vi "REPORT - Autofrettage.vi"(8 "error in (no error)":errorcluster, 10 "Report Save Path":path, 11 "TDMS file path":path) -> ()   [LabVIEW 2025]
uses:
  <vilib>/printing/EasyPrintingControls.llb/contents.ctl
  <vilib>/Utility/NIReport.llb/Report Type (with Quick Print).ctl
  <vilib>/Utility/error.llb/Trim Whitespace One-Sided.vi
  <vilib>/printing/EasyPrinting.llb/Print VI Panel or Documentation (path).vi
  <vilib>/Utility/NIReport.llb/NI_report.lvclass
  <vilib>/Utility/NIReport.llb/NI_ReportGenerationCore.lvlib
panel:
  in  "Close":bool
  in  "PRINT REPORT":bool
  out "graph":cluster{"X":dbl[], "Y":dbl[]}[](graph)
  out "Operator:":string
  out "String":string
  in  "Comments:":string
  out "Test Date:":dbl format="%<%x>T"
  out "Test ID:":string
  out "Part Number:":string
  out "Job Number:":string
  # "Autofrettage Run Report"
  # "Unit Under Test"
  # "Pressure v. Time"
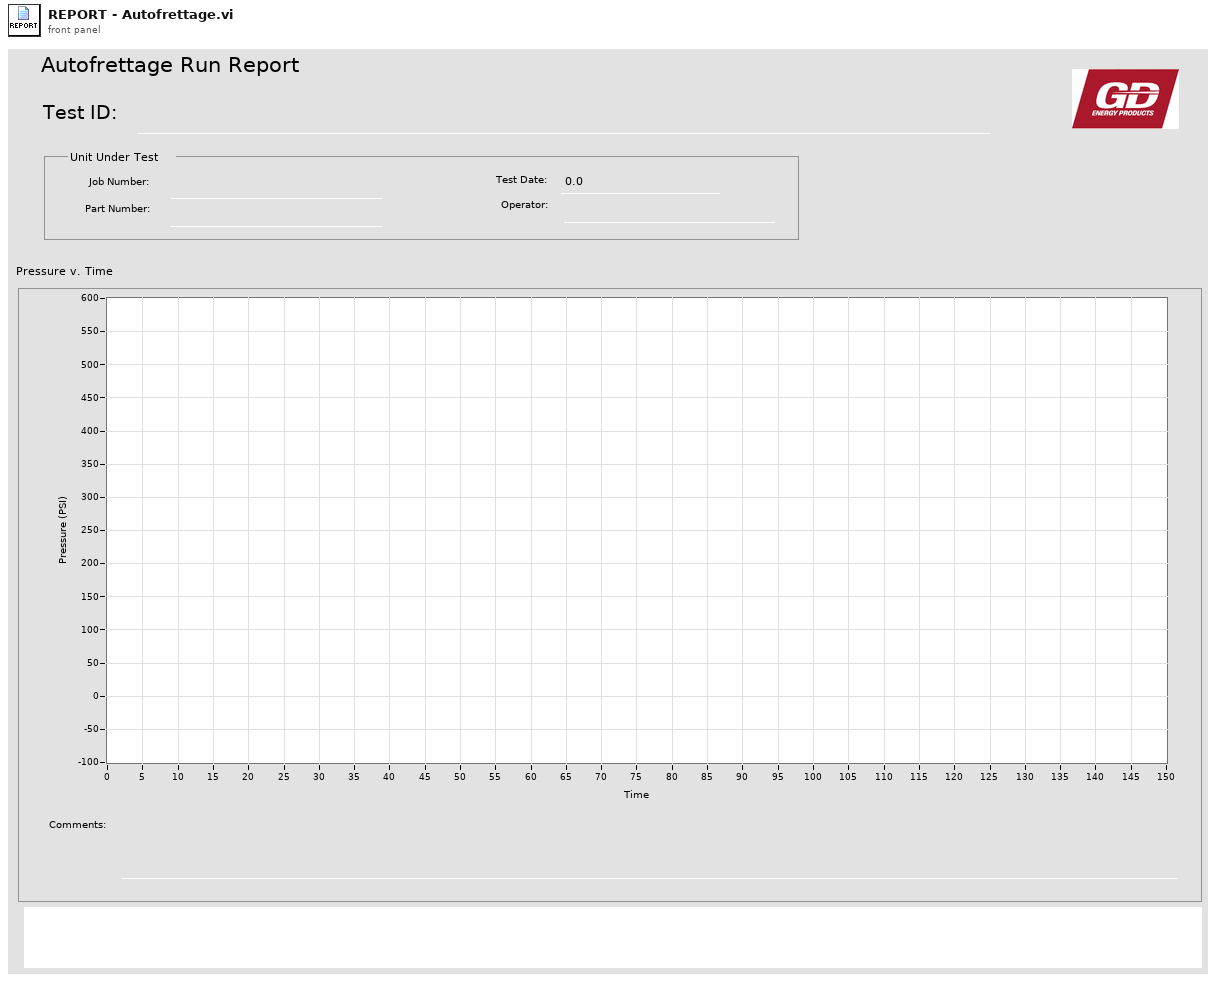
[diagram p1: front panel]
types:
  T1 = typedef "NI_ReportGenerationCore.lvlib/Report Type (with Quick Print).ctl" = enum16{"Quick Print", "HTML", "Word", "Excel"}
  T2 = typedef "NI_ReportGenerationCore.lvlib/contents.ctl" = u16
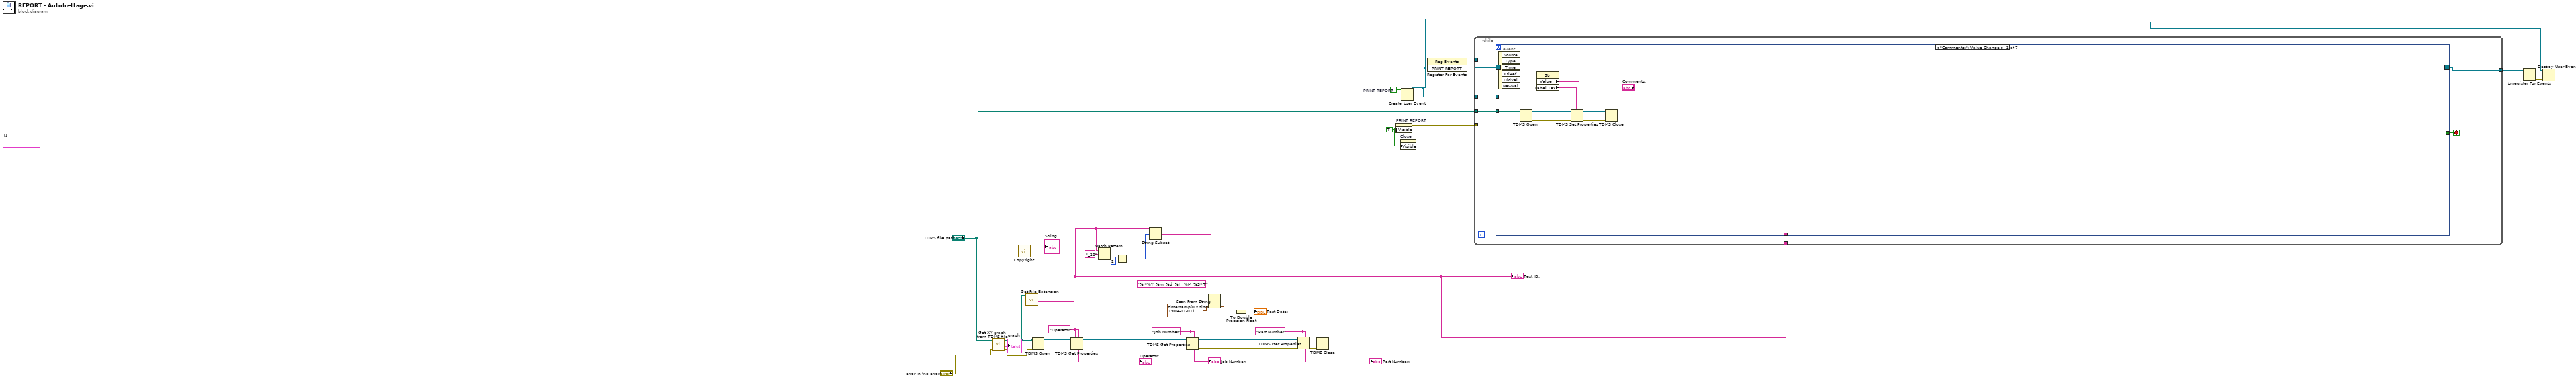
[diagram p0: block diagram]
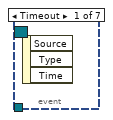
[diagram p2: hidden frame]
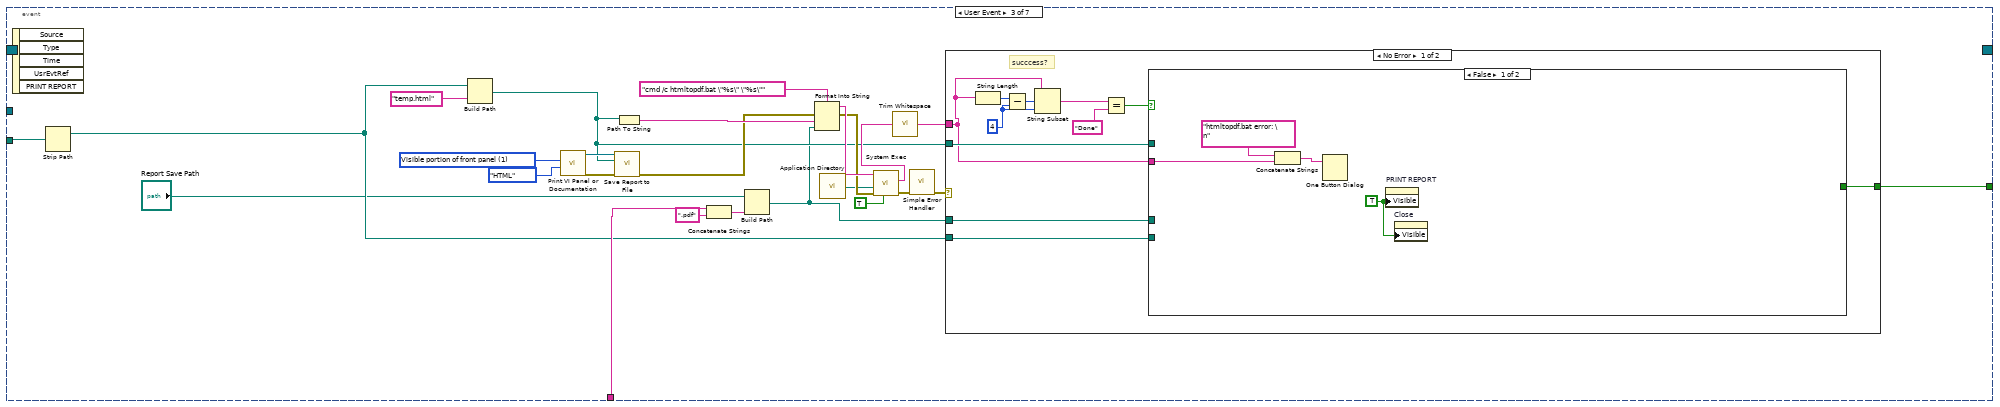
[diagram p3: hidden frame]
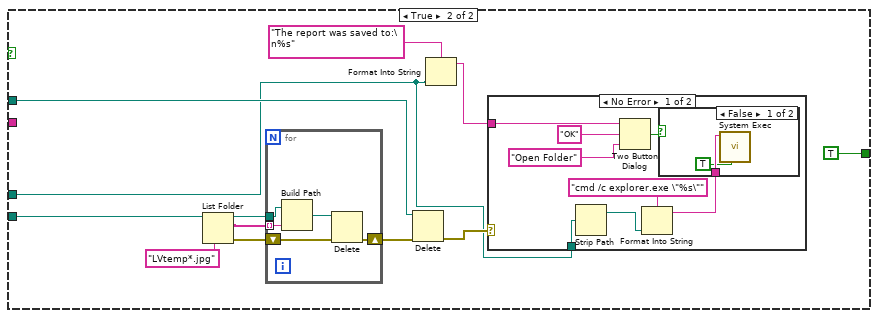
[diagram p4: hidden frame]
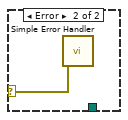
[diagram p6: hidden frame]
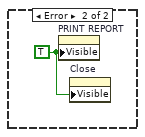
[diagram p7: hidden frame]
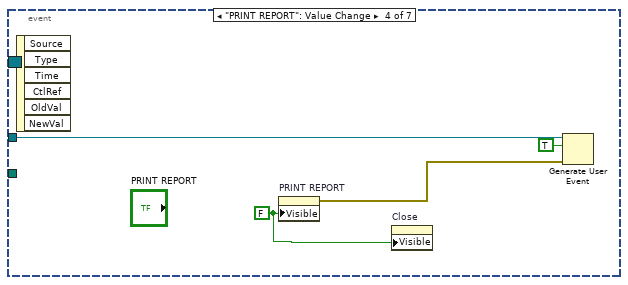
[diagram p8: hidden frame]
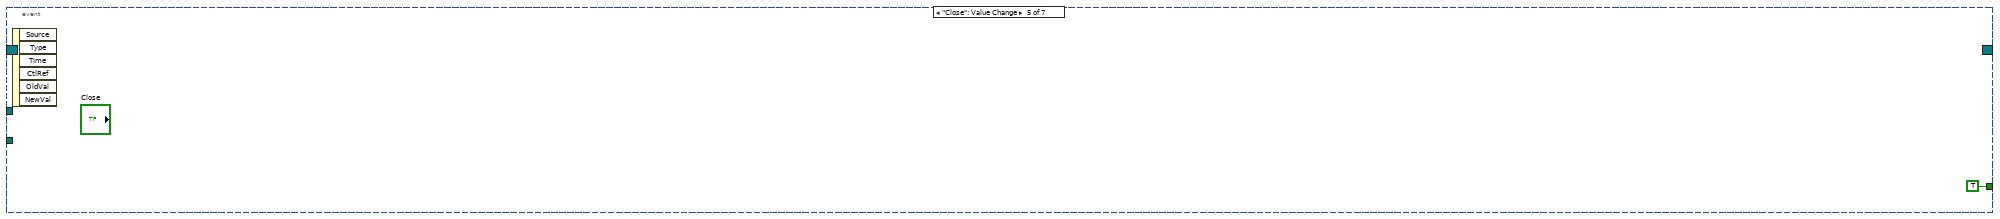
[diagram p9: hidden frame]
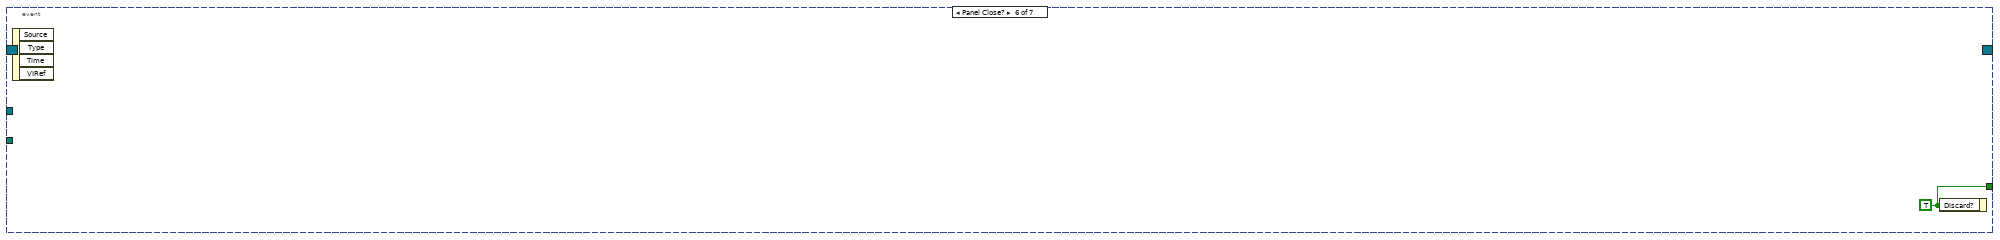
[diagram p10: hidden frame]
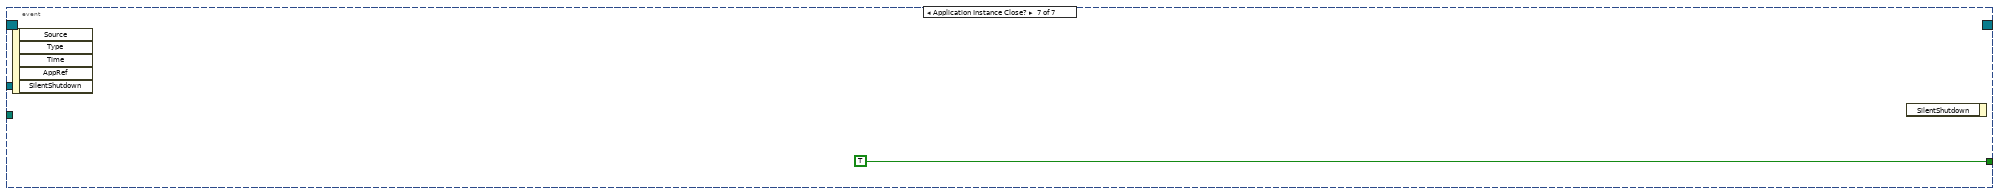
[diagram p11: hidden frame]
diagram:
  w10 = TRUE ("Visible")
  w16 = TRUE  # PRINT REPORT
  w23 = "Part Number" ("channel name")
  w25 = "Job Number" ("channel name")
  w21 = "Operator" ("channel name")
  (unwired) cluster{"X":dbl[], "Y":dbl[]}[] [] ("Restoring Force")
  n1 = call "Get XY graph from TDMS file.vi"("error in"="error in (no error)", "TDMS file path"="TDMS file path") -> ("error out"=w8:errorcluster, "graph"=→"graph":cluster{"X":dbl[], "Y":dbl[]}[], "TDMS file path out"=w7:path)  [unwired: 7 in]
  n2 = call "Copyright.vi"() -> ("String"=→"String":string)  [unwired: 11 in]
  n3 = call <vilib>:"Get File Extension.vi"("file"=w7) -> ("filename without extension"=w2:string)  [unwired: 6 in, 4 out]
  "Test ID:" <- w2
  n4 = TDMS Open(8:w8, 11:w7) -> (0:w30:errorcluster, 3:w35:refnum<k34>)  [unwired: 5 in]
  n5 = TDMS Get Properties(5:w21, 7:w21, 8:w30, 11:w35) -> (0:w31:errorcluster, 3:w34:refnum<k34>, 4:→"Operator:":string)  [unwired: 2 in, 3 out]
  n6 = Match Pattern(string=w2, regular expression="_20") -> (offset past match=w5:i32)  [unwired: 1 in, 3 out]
  n7 = Subtract(x=w5, y=2) -> (x-y=w3:i32)
  n8 = String Subset(string=w2, offset (0)=w3) -> (substring=w1:string)  [unwired: 1 in]
  n9 = TDMS Get Properties(5:w25, 7:w25, 8:w31, 11:w34) -> (0:w32:errorcluster, 3:w33:refnum<k34>, 4:→"Job Number:":string)  [unwired: 2 in, 3 out]
  n10 = Scan From String(format string="%<%Y_%m_%d_%H_%M_%S>T", input string=w1, default 1=timestamp(0 s since 1904-01-01)) -> (output 1=w27:timestamp)  [unwired: 2 in, 3 out]
  n11 = To Double Precision Float(number=w27) -> (double precision float=→"Test Date:":dbl)
  n12 = TDMS Get Properties(5:w23, 7:w23, 8:w32, 11:w33) -> (0:w18:errorcluster, 3:w17:refnum<k34>, 4:→"Part Number:":string)  [unwired: 2 in, 3 out]
  n13 = TDMS Close(8:w18, 11:w17) -> ()  [unwired: 2 out]
  n14 = property on="PRINT REPORT" class="Bool"("Visible"=w10) -> (error out=w11:errorcluster)  [unwired: 2 in, 1 out]
  n15 = property on="Close" class="Bool"("Visible"=w10) -> ()  [unwired: 2 in, 2 out]
  n16 = Create User Event(user event datatype=w16) -> (user event=w12:refnum<user-event>)  [unwired: 1 in, 1 out]
  n17 = register-events(w12) -> (reference out=w15:refnum<event-registration>)  [unwired: 2 in, 1 out]
  n18 = while {
    tunnel: "TDMS file path" -> [w42]
    tunnel: w2 -> [w41]
    tunnel: w15 -> [w40]
    tunnel: w12 -> [w39]
    tunnel: [w38] -> w14
    tunnel: w11 -> [_]
    stop <- w43 stop-if-true
    n19 = event shown="[1] \"Comments:\": Value Change" {
      selector: w40 -> [_ _ _ _ _ _ _]
      dyn-events: [_ _ _ _ _ _ _] -> w38
      timeout: _ -> [_ _ _ _ _ _ _]
      tunnel: [_ _ w73 _ TRUE ("Discard?") w126 TRUE] -> w43
      tunnel: w42 -> [_ w51 w75 _ _ _ _]
      tunnel: w41 -> [_ _ w76 _ _ _ _]
      tunnel: w39 -> [_ _ _ w124 _ _ _]
      event Timeout {
        n20 = event-data() -> ()  [unwired: 1 in, 3 out]
      }
      event "Comments:": Value Change {
        n21 = event-data() -> ("CtlRef"=w49:refnum<vi>)  [unwired: 1 in, 5 out]
        n22 = TDMS Open(11:w51) -> (0:w44:errorcluster, 3:w50:refnum<k34>)  [unwired: 6 in]
        n23 = property class="Str"(reference=w49) -> ("Value"=w46:string, "Label.Text"=w47:string)  [unwired: 1 in, 2 out]
        n24 = TDMS Set Properties(5:w46, 7:w47, 8:w44, 11:w50) -> (0:w45:errorcluster, 3:w48:refnum<k34>)  [unwired: 2 in, 2 out]
        n25 = TDMS Close(8:w45, 11:w48) -> ()  [unwired: 2 out]
      }
      event User Event {
        w67 = T2 1 items=["Complete front panel", "Visible portion of front panel", "Icon, description, panel and diagram", "Documentation: Using the panel", "Documentation: Using as a subVI", "Documentation: Complete", "Documentation: Custom"] ("contents (complete front panel)")
        n26 = event-data() -> ()  [unwired: 1 in, 5 out]
        n27 = Strip Path(path=w75) -> (stripped path=w74:path)  [unwired: 1 out]
        n28 = Build Path(base path=w74, name or relative path="temp.html" ("string")) -> (appended path=w56:path)
        n29 = call-poly <vilib>:"Print VI Panel or Documentation.vi"("report type (Quick Print)"=Report_Type_(with_Quick_Print)."HTML", "contents (complete front panel)"=w67) -> ("error out"=w64:errorcluster, "report out"=w70:refnum<class "NI_report.lvclass">)  [unwired: 8 in]
        n30 = call-dynamic "Save Report to File.vi"("report in"=w70, "report file path"=w56, "error in (no error)"=w64) -> ("error out"=w60:errorcluster)  [unwired: 11 in, 1 out]
        n31 = Path To String(path=w56) -> (string=w71:string)
        n32 = Concatenate Strings(w76, ".pdf" ("string")) -> (w62:string)
        n33 = Build Path(base path="Report Save Path", name or relative path=w62) -> (appended path=w54:path)
        n34 = Format Into String(format string="cmd /c htmltopdf.bat \"%s\" \"%s\"" ("command line"), error in=w60, w71, w54) -> (resulting string=w72:string, error out=w65:errorcluster)  [unwired: 1 in]
        n35 = call <vilib>:"Application Directory.vi"() -> ("Application Directory"=w55:path)
        n36 = call <vilib>:"System Exec.vi"("run minimized? (F)"=TRUE, "error in (no error)"=w65, "working directory"=w55, "command line"=w72) -> ("error out"=w66:errorcluster, "standard error"=w58:string)  [unwired: 4 in, 2 out]
        n37 = call <vilib>:"Trim Whitespace.vi"("string"=w58) -> ("trimmed string"=w52:string)  [unwired: 1 in]
        n38 = call <vilib>:"Simple Error Handler.vi"("error in (no error)"=w66) -> ("error out"=w59:errorcluster)  [unwired: 4 in, 4 out]
        n39 = case shown="No Error" w59 {
          tunnel: w74 -> [w87 _]
          tunnel: w56 -> [w86 _]
          tunnel: w52 -> [w77 _]
          tunnel: [w85 _] -> w73
          tunnel: w54 -> [w84 _]
          frame No Error {
            w81 = 4 ("y")
            # "succcess?"
            n40 = String Length(string=w77) -> (length=w83:i32)
            n41 = Subtract(x=w83, y=w81) -> (x-y=w82:i32)
            n42 = String Subset(string=w77, offset (0)=w82, length (rest)=w81) -> (substring=w80:string)
            n43 = Equal?(x=w80, y="Done") -> (x = y?=w78:bool)
            n44 = case shown="False" w78 {
              tunnel: w87 -> [_ w103]
              tunnel: w86 -> [_ w102]
              tunnel: w77 -> [w90 _]
              tunnel: [_ TRUE] -> w85
              tunnel: w84 -> [_ w97]
              frame False {
                w91 = TRUE ("Visible")
                n45 = Concatenate Strings("htmltopdf.bat error: \n" ("string"), w90) -> (w89:string)
                n46 = One Button Dialog(message=w89) -> ()  [unwired: 1 in, 1 out]
                n47 = property on="PRINT REPORT" class="Bool"("Visible"=w91) -> ()  [unwired: 2 in, 2 out]
                n48 = property on="Close" class="Bool"("Visible"=w91) -> ()  [unwired: 2 in, 2 out]
              }
              frame True {
                n49 = List Folder(path=w103, pattern="LVtemp*.jpg") -> (path out=w94:path, filenames=w95:string[], error out=w92:errorcluster)  [unwired: 2 in, 1 out]
                n50 = for {
                  tunnel: w95 -> [w108] mode=indexing
                  tunnel: w94 -> [w107]
                  shift-right: [w105] -> w93
                  shift-left: w92 -> [w104]
                  n51 = Build Path(base path=w107, name or relative path=w108) -> (appended path=w106:path)
                  n52 = Delete(path (use dialog)=w106, error in=w104) -> (error out=w105:errorcluster)  [unwired: 3 in, 2 out]
                }
                n53 = Delete(path (use dialog)=w102, error in=w93) -> (error out=w98:errorcluster)  [unwired: 3 in, 2 out]
                n54 = Format Into String(format string="The report was saved to:\n%s", w97) -> (resulting string=w99:string)  [unwired: 2 in, 1 out]
                n55 = case shown="No Error" w98 {
                  selector: w98 -> [_ w119]
                  tunnel: w99 -> [w116 _]
                  tunnel: w97 -> [w110 _]
                  frame No Error {
                    n56 = Strip Path(path=w110) -> (stripped path=w109:path)  [unwired: 1 out]
                    n57 = Two Button Dialog(message=w116, 1:"Open Folder" ("F button name (\"Cancel\")"), 2:"OK" ("T button name (\"OK\")")) -> (T button?=w114:bool)
                    n58 = Format Into String(format string="cmd /c explorer.exe \"%s\"", w109) -> (resulting string=w112:string)  [unwired: 2 in, 1 out]
                    n59 = case shown="False" w114 {
                      tunnel: w112 -> [w118 _]
                      frame False {
                        n60 = call <vilib>:"System Exec.vi"("run minimized? (F)"=TRUE, "command line"=w118) -> ()  [unwired: 6 in, 4 out]
                      }
                      frame True {
                      }
                    }
                  }
                  frame Error {
                    n61 = call <vilib>:"Simple Error Handler.vi"("error in (no error)"=w119) -> ()  [unwired: 4 in, 5 out]
                  }
                }
              }
            }
          }
          frame Error {
            w120 = TRUE ("Visible")
            n62 = property on="PRINT REPORT" class="Bool"("Visible"=w120) -> ()  [unwired: 2 in, 2 out]
            n63 = property on="Close" class="Bool"("Visible"=w120) -> ()  [unwired: 2 in, 2 out]
          }
        }
      }
      event "PRINT REPORT": Value Change {
        w122 = FALSE ("Visible")
        n64 = event-data() -> ()  [unwired: 1 in, 6 out]
        n65 = property on="PRINT REPORT" class="Bool"("Visible"=w122) -> (error out=w123:errorcluster)  [unwired: 2 in, 1 out]
        n66 = property on="Close" class="Bool"("Visible"=w122) -> ()  [unwired: 2 in, 2 out]
        n67 = Generate User Event(user event=w124, event data cluster=TRUE ("event data"), error in=w123) -> ()  [unwired: 1 in, 2 out]
      }
      event "Close": Value Change {
        n68 = event-data() -> ()  [unwired: 1 in, 6 out]
      }
      event Panel Close? {
        w126 = TRUE ("Discard?")
        n69 = event-data() -> ()  [unwired: 1 in, 4 out]
        n70 = event-data("Discard?"=w126) -> ()  [unwired: 1 in, 1 out]
      }
      event Application Instance Close? {
        n71 = event-data() -> ()  [unwired: 1 in, 5 out]
        n72 = event-data() -> ()  [unwired: 2 in, 1 out]
      }
    }
  }
  n73 = Unregister For Events(event registration refnum=w14) -> (error out=w13:errorcluster)  [unwired: 1 in]
  n74 = Destroy User Event(user event=w12, error in=w13) -> ()  [unwired: 1 out]
